vi "Add WCM value.vi"(8 "error in (no error)":errorcluster, 10 "WCM value":sgl, 11 "Experiment in":refnum<class "Experiment.lvclass">) -> (0 "error out":errorcluster, 3 "Experiment out":refnum<class "Experiment.lvclass">)   [LabVIEW 2015, in "Experiment.lvclass"]
uses:
  Experiment.lvclass
  Experiment.lvclass/Experiment.ctl
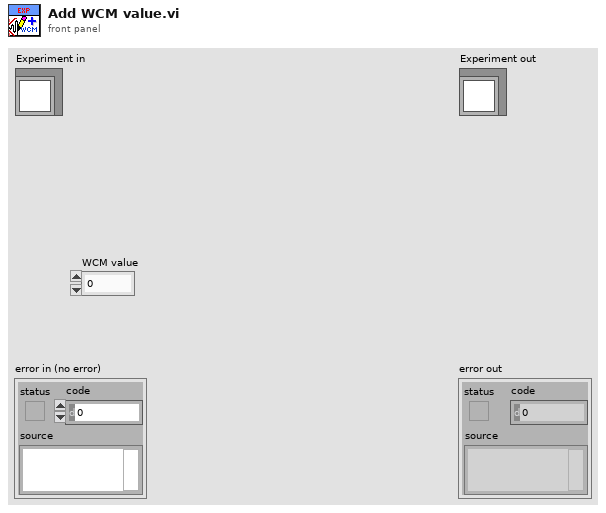
[diagram p1: front panel]
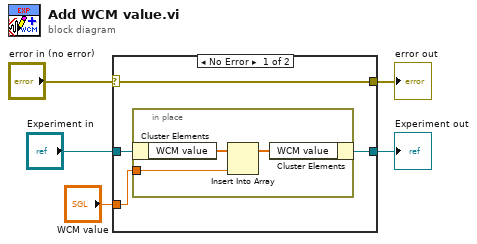
[diagram p0: block diagram]
diagram:
  n1 = case shown="No Error" "error in (no error)" {
    selector: "error in (no error)" -> [w9 w13]
    tunnel: [w9 w13] -> w4
    tunnel: [w6 w14] -> w2
    tunnel: "Experiment in" -> [w8 w14]
    tunnel: "WCM value" -> [w7 _]
    frame No Error {
      n2 = in-place {
        in-place-border: w7 -> [w10]
        n3 = in-place-cluster #1(w8) -> ("WCM value"=w12:sgl[])
        n4 = Insert Into Array(array=w12, new element=w10) -> (w11:sgl[])  [unwired: 1 in]
        n5 = in-place-cluster #1("WCM value"=w11) -> (w6:refnum<class "Experiment.lvclass">)
      }
    }
    frame Error {
    }
  }
  "error out" <- w4
  "Experiment out" <- w2
